vi "Digital Write Multiple Channels.vi"(8 "error in (no error)":errorcluster, 9 "Values":bool[](array[boolean]), 10 "Indices":i32[](array[numeric]), 11 "NI-DAQ in":refnum<class "NI-DAQ.lvclass">) -> (0 "error out":errorcluster, 3 "NI-DAQ out":refnum<class "NI-DAQ.lvclass">)   [LabVIEW 2016, in "NI-DAQ.lvclass"]
uses:
  NI-DAQ.lvclass
  NI-DAQ.lvclass/NI-DAQ.ctl
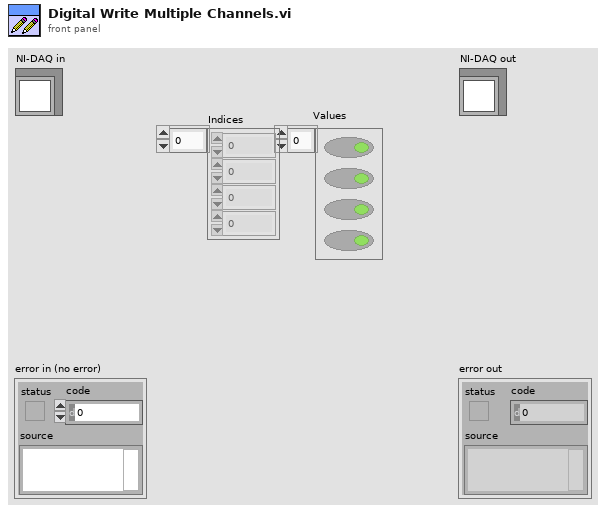
[diagram p1: front panel]
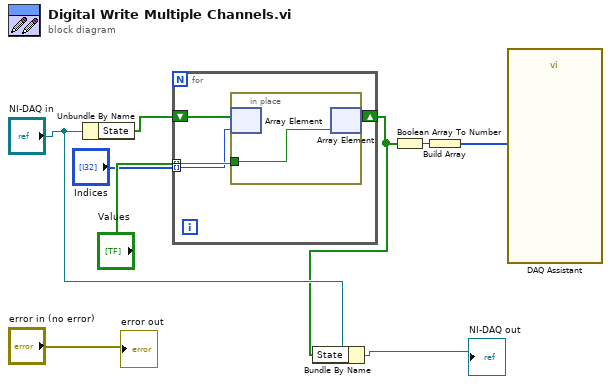
[diagram p0: block diagram]
diagram:
  n1 = Unbundle By Name("NI-DAQ in") -> ("State"=w2:bool[])
  n2 = for {
    tunnel: "Values" -> [w13] mode=indexing
    tunnel: "Indices" -> [w12] mode=indexing
    shift-right: [w10] -> w1
    shift-left: w2 -> [w11]
    n3 = in-place {
      in-place-border: w13 -> [w14]
      n4 = in-place-array #1(w11, w12) -> ()  [unwired: 1 out]
      n5 = in-place-array #1(w14) -> (w10:bool[])  [unwired: 1 out]
    }
  }
  n6 = Bundle By Name(cluster="NI-DAQ in", "State"=w1) -> (→"NI-DAQ out":refnum<class "NI-DAQ.lvclass">)
  n7 = Boolean Array To Number(Boolean array=w1) -> (number=w8:u32)
  n8 = Build Array(w8) -> (w7:u32[])
  n9 = call "DAQ Assistant"("data"=w7) -> ()  [unwired: 17 in, 2 out]
  "error out" <- "error in (no error)"
